vi "HSMS Release.vi"(8 "error in (no error)":errorcluster, 11 "HSMS Class in":refnum<class "HSMS Class.lvclass">) -> (0 "error out":errorcluster)   [LabVIEW 2020, in "SECS Communication.lvlib" / "HSMS Class.lvclass"]
uses:
  HSMS Class.lvclass
  HSMS Class.lvclass/HSMS Class.ctl
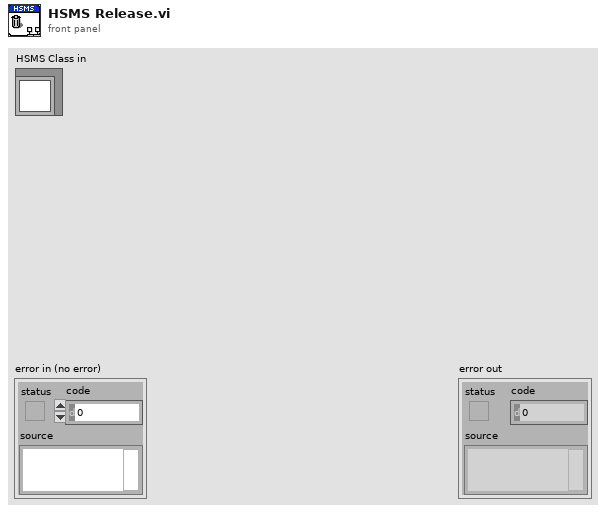
[diagram p1: front panel]
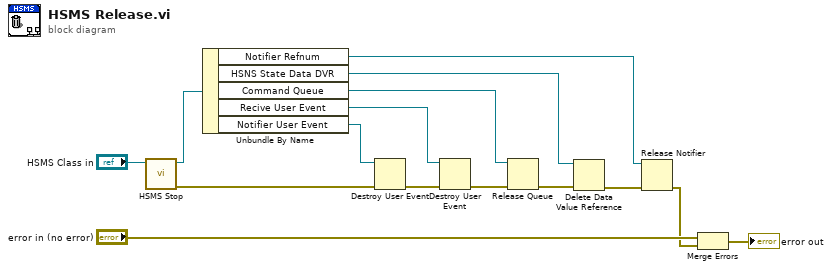
[diagram p0: block diagram]
diagram:
  n1 = call "HSMS Stop.vi"("HSMS Class in"="HSMS Class in") -> ("error out"=w2:errorcluster, "HSMS Class out"=w1:refnum<class "HSMS Class.lvclass">)  [unwired: 9 in]
  n2 = Unbundle By Name(w1) -> ("Notifier Refnum"=w15:refnum<notifier>, "HSNS State Data DVR"=w13:refnum<data-value>, "Command Queue"=w10:refnum<queue>, "Recive User Event"=w12:refnum<user-event>, "Notifier User Event"=w4:refnum<user-event>)
  n3 = Destroy User Event(user event=w4, error in=w2) -> (error out=w5:errorcluster)
  n4 = Destroy User Event(user event=w12, error in=w5) -> (error out=w11:errorcluster)
  n5 = Release Queue(queue=w10, error in (no error)=w11) -> (error out=w9:errorcluster)  [unwired: 1 in, 2 out]
  n6 = Delete Data Value Reference(data value reference=w13, error in=w9) -> (error out=w14:errorcluster)  [unwired: 1 out]
  n7 = Release Notifier(notifier=w15, error in (no error)=w14) -> (error out=w6:errorcluster)  [unwired: 1 in, 2 out]
  n8 = Merge Errors("error in (no error)", w6) -> (→"error out":errorcluster)
